vi "WebCAM_Init2.vi"(8 "error in (no error)":errorcluster, 10 "PictureBox":refnum<k24>, 11 "Window Title":string="Title") -> (0 "error out":errorcluster, 1 "return type":u32, 2 "error initialising":bool, 3 "window handle":u32)   [LabVIEW 2011]
uses:
  System.Windows.Forms
  user32.dll
  avicap32.dll
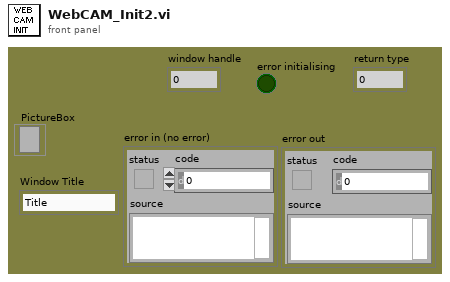
[diagram p1: front panel]
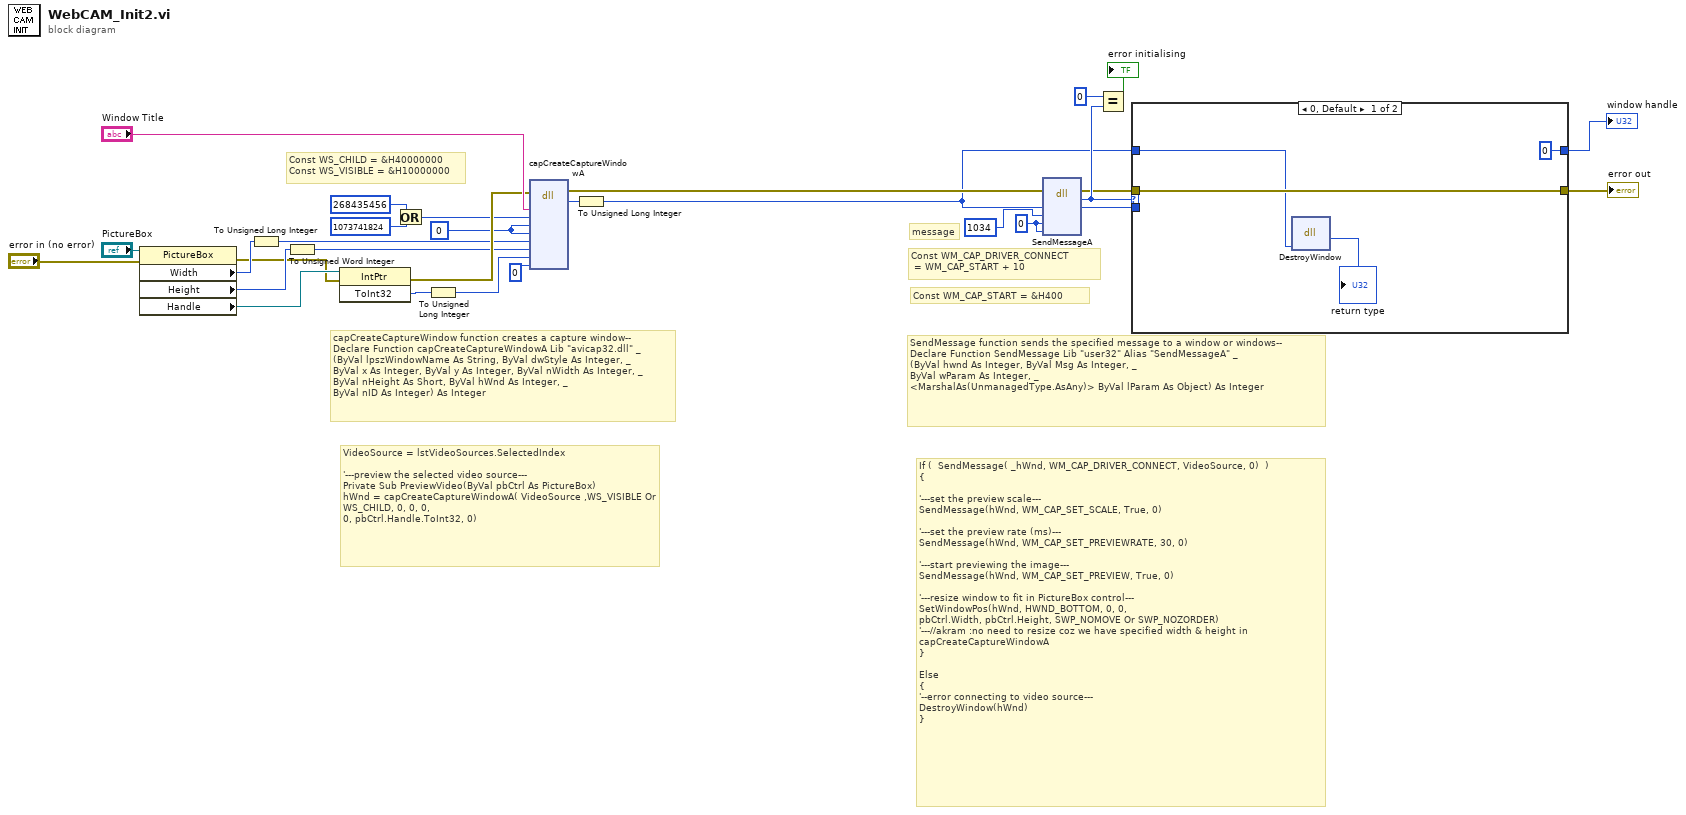
[diagram p0: block diagram]
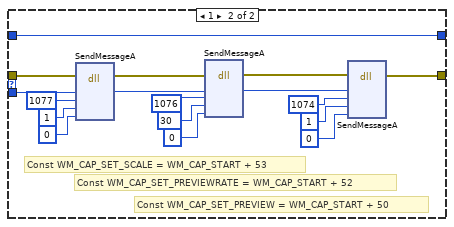
[diagram p2: hidden frame]
diagram:
  w11 = u32 0 ("wParam")
  w14 = u32 0 ("y")
  # "If (  SendMessage( _hWnd, WM_CAP_DRIVER_CONNECT, VideoSource, 0)  )\n{\n\n'---set the preview scale---\nSendMessage(hWnd, WM_CAP_SET_SCALE, True, 0)\n\n'---set the preview rate (ms)---\nSendMessage(hWnd, WM_CAP_SET_PREVIEWRATE, 30, 0)\n\n'---start previewing the image---\nSendMessage(hWnd, WM_CAP_SET_PREVIEW, True, 0)\n\n'---resize window to fit in PictureBox control---\nSetWindowPos(hWnd, HWND_BOTTOM, 0, 0, \npbCtrl.Width, pbCtrl.Height, SWP_NOMOVE Or SWP_NOZORDER)\n'---//akram :no need to resize coz we have specified width & height in capCreateCaptureWindowA\n}\n\nElse\n{\n'--error connecting to video source---\nDestroyWindow(hWnd)\n}"
  # "Const WM_CAP_START = &H400"
  # "Const WM_CAP_DRIVER_CONNECT\n = WM_CAP_START + 10"
  # "VideoSource = lstVideoSources.SelectedIndex\n\n'---preview the selected video source---\nPrivate Sub PreviewVideo(ByVal pbCtrl As PictureBox)\nhWnd = capCreateCaptureWindowA( VideoSource ,WS_VISIBLE Or WS_CHILD, 0, 0, 0, \n0, pbCtrl.Handle.ToInt32, 0)"
  # "message"
  # "SendMessage function sends the specified message to a window or windows--\nDeclare Function SendMessage Lib \"user32\" Alias \"SendMessageA\" _\n(ByVal hwnd As Integer, ByVal Msg As Integer, _\nByVal wParam As Integer, _\n<MarshalAs(UnmanagedType.AsAny)> ByVal lParam As Object) As Integer"
  # "capCreateCaptureWindow function creates a capture window--\nDeclare Function capCreateCaptureWindowA Lib \"avicap32.dll\" _\n(ByVal lpszWindowName As String, ByVal dwStyle As Integer, _\nByVal x As Integer, ByVal y As Integer, ByVal nWidth As Integer, _\nByVal nHeight As Short, ByVal hWnd As Integer, _\nByVal nID As Integer) As Integer"
  # "Const WS_CHILD = &H40000000\nConst WS_VISIBLE = &H10000000"
  n1 = property class="PictureBox"(reference="PictureBox", error in="error in (no error)") -> (error out=w23:errorcluster, "Width"=w25:i32, "Height"=w26:i32, "Handle"=w24:refnum<k24>)  [unwired: 1 out]
  n2 = To Unsigned Long Integer(number=w25) -> (unsigned 32bit integer=w22:u32)
  n3 = To Unsigned Word Integer(number=w26) -> (unsigned 16bit integer=w20:u16)
  n4 = invoke class="IntPtr" method="ToInt32"(reference=w24, error in=w23) -> (error out=w27:errorcluster, "ToInt32"=w15:i32)  [unwired: 1 in, 1 out]
  n5 = Or(x=u32 268435456, y=u32 1073741824) -> (x .or. y?=w18:u32)
  n6 = To Unsigned Long Integer(number=w15) -> (unsigned 32bit integer=w21:u32)
  n7 = dll-call lib="avicap32.dll" fn="capCreateCaptureWindowA"(error in=w27, "lpszWindowName"="Window Title", "dwStyle"=w18, "x"=w14, "y"=w14, "nWidth"=w22, "nHeight"=w20, "hwnd"=w21, "nID"=u32 0) -> (error out=w7:errorcluster, "return type"=w9:i32)  [unwired: 10 in, 1 out]
  n8 = To Unsigned Long Integer(number=w9) -> (unsigned 32bit integer=w4:u32)
  n9 = dll-call lib="user32.dll" fn="SendMessageA"(error in=w7, "hwnd"=w4, "msg"=u32 1034, "wParam"=w11, "lparam"=w11) -> (error out=w6:errorcluster, "return type"=w10:u32, "hwnd"=w8:u32)  [unwired: 5 in, 1 out]
  n10 = Equal?(x=u32 0, y=w10) -> (x = y?=→"error initialising":bool)
  n11 = case shown="0, Default" w10 {
    tunnel: w8 -> [_ w50]
    tunnel: w6 -> [w33 w36]
    tunnel: [w33 w35] -> w28
    tunnel: w4 -> [w31 w34]
    tunnel: [u32 0 w34] -> w3
    frame 0, Default {
      n12 = dll-call lib="user32.dll" fn="DestroyWindow"("hwnd"=w31) -> ("return type"=→"return type":u32)  [unwired: 4 in, 2 out]
    }
    frame 1 {
      # "Const WM_CAP_SET_PREVIEW = WM_CAP_START + 50"
      # "Const WM_CAP_SET_PREVIEWRATE = WM_CAP_START + 52"
      # "Const WM_CAP_SET_SCALE = WM_CAP_START + 53"
      n13 = dll-call lib="user32.dll" fn="SendMessageA"(error in=w36, "hwnd"=w50, "msg"=u32 1077, "wParam"=u32 1 ("msg"), "lparam"=u32 0 ("msg")) -> (error out=w43:errorcluster, "hwnd"=w42:u32)  [unwired: 6 in, 1 out]
      n14 = dll-call lib="user32.dll" fn="SendMessageA"(error in=w43, "hwnd"=w42, "msg"=u32 1076, "wParam"=u32 30 ("msg"), "lparam"=u32 0 ("msg")) -> (error out=w38:errorcluster, "hwnd"=w37:u32)  [unwired: 6 in, 1 out]
      n15 = dll-call lib="user32.dll" fn="SendMessageA"(error in=w38, "hwnd"=w37, "msg"=u32 1074, "wParam"=u32 1 ("msg"), "lparam"=u32 0 ("msg")) -> (error out=w35:errorcluster)  [unwired: 7 in, 1 out]
    }
  }
  "error out" <- w28
  "window handle" <- w3
